vi "Right Visible.vi"(8 "Current column":i32, 9 "Current row":i32, 10 "Full array":i32[][](array[numeric]), 11 "Element":i32) -> (2 "Viewing Distance":i32, 3 "Visible":bool)   [LabVIEW 2021]
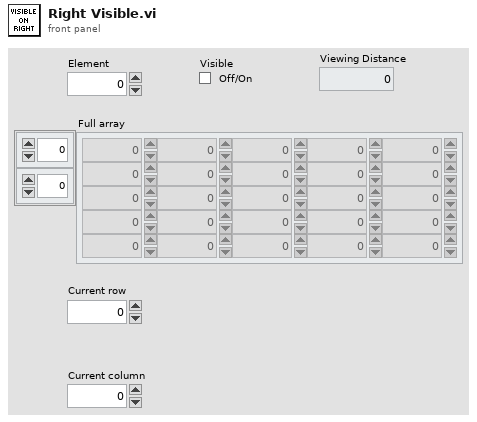
[diagram p1: front panel]
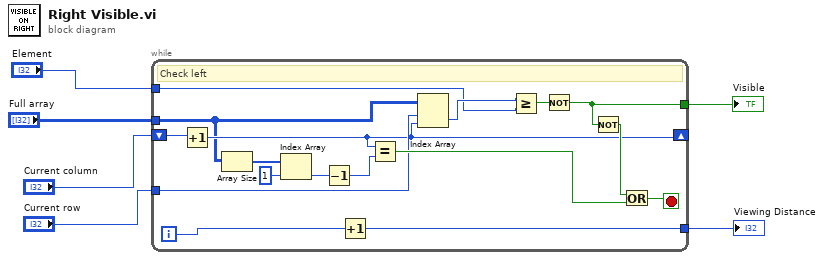
[diagram p0: block diagram]
diagram:
  n1 = while {
    shift-right: [w18] -> _
    shift-left: "Current column" -> [w19]
    tunnel: "Element" -> [w10]
    tunnel: "Full array" -> [w17]
    tunnel: "Current row" -> [w20]
    tunnel: [w9] -> w6
    tunnel: [w7] -> w1
    i -> [w8]
    stop <- w21 stop-if-true
    # "Check left"
    n2 = Increment(x=w19) -> (x+1=w18:i32)
    n3 = Array Size(array=w17) -> (size(s)=w16:i32[])
    n4 = Index Array(array=w16, index=1) -> (element=w15:i32)
    n5 = Decrement(x=w15) -> (x-1=w14:i32)
    n6 = Increment(x=w8) -> (x+1=w7:i32)
    n7 = Equal?(x=w18, y=w14) -> (x = y?=w22:bool)
    n8 = Index Array(array=w17, index (row)=w20, index (col)=w18) -> (element=w11:i32)
    n9 = Greater Or Equal?(x=w11, y=w10) -> (x >= y?=w12:bool)
    n10 = Not(x=w12) -> (.not. x?=w9:bool)
    n11 = Not(x=w9) -> (.not. x?=w23:bool)
    n12 = Or(x=w23, y=w22) -> (x .or. y?=w21:bool)
  }
  "Visible" <- w6
  "Viewing Distance" <- w1
